vi "Clase5b.vi"() -> ()   [LabVIEW 2011]
panel:
  out "Aceptado":bool
  out "Edad":dbl
  in  "Experiencia":u16(ring) items=["Experiencia", "No tiene experiencia"]
  in  "Tiene titulo":u16(ring) items=["No tiene", "Tiene"]
  # "Se debe seleccionar si tiene o no tiene titulo, luego si tiene experiencia y generar a la edad\nentre 20 y 70.\n\nEs contratado si la edad es mayor a 25 y si"
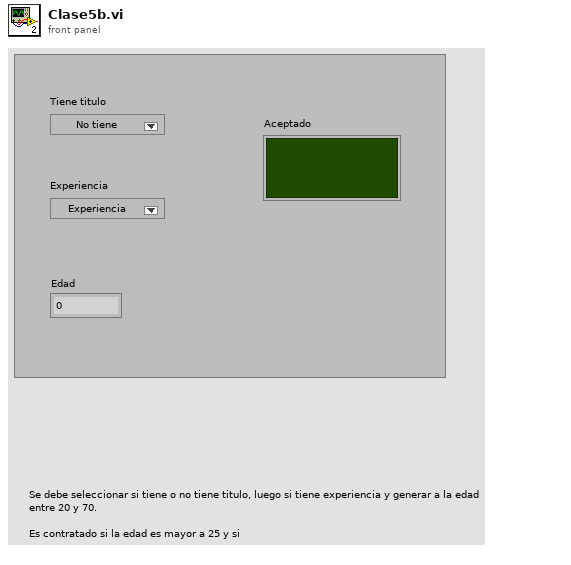
[diagram p1: front panel]
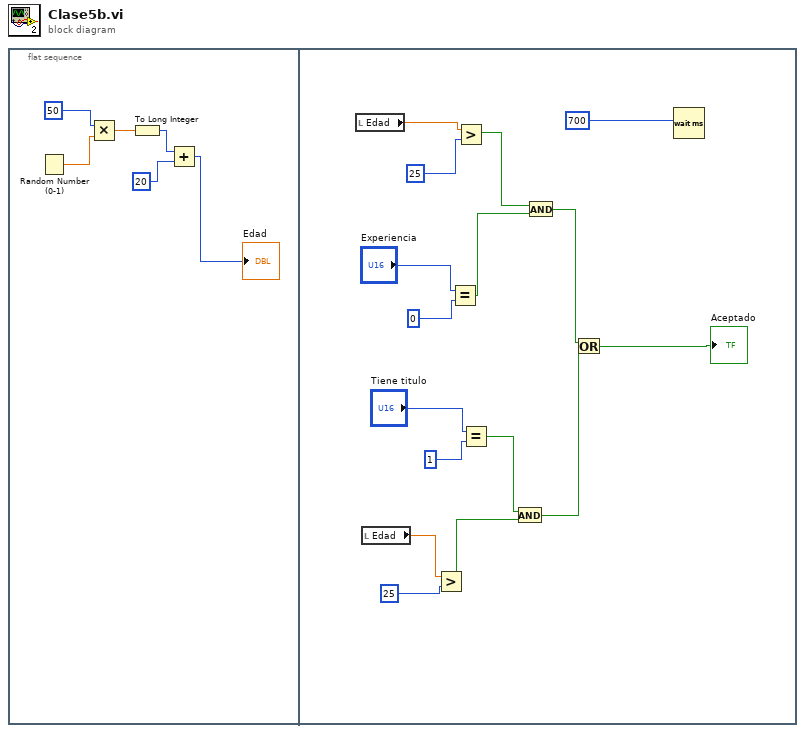
[diagram p0: block diagram]
diagram:
  n1 = flat-sequence {
    frame #0 {
      n2 = Random Number (0-1)() -> (number: 0 to 1=w5:dbl)
      n3 = Multiply(x=50, y=w5) -> (x*y=w4:dbl)
      n4 = To Long Integer(number=w4) -> (32bit integer=w3:i32)
      n5 = Add(x=w3, y=20) -> (x+y=→"Edad":i32)
    }
    frame #1 {
      n6 = local read "Edad"() -> (w22:dbl)
      n7 = local read "Edad"() -> (w14:dbl)
      n8 = Greater?(x=w14, y=25) -> (0:w12:bool)
      n9 = Equal?(x="Experiencia", y=0) -> (x = y?=w17:bool)
      n10 = Greater?(x=w22, y=25) -> (0:w18:bool)
      n11 = Equal?(x="Tiene titulo", y=1) -> (x = y?=w11:bool)
      n12 = And(x=w11, y=w12) -> (x .and. y?=w10:bool)
      n13 = And(x=w18, y=w17) -> (x .and. y?=w9:bool)
      n14 = Or(x=w9, y=w10) -> (x .or. y?=→"Aceptado":bool)
      n15 = Wait (ms)(milliseconds to wait=700) -> ()  [unwired: 1 out]
    }
  }
